vi "未命名 3.vi"() -> ()   [LabVIEW 2015]
uses:
  <vilib>/Utility/config.llb/Write Key (String).vi
  <vilib>/Utility/config.llb/Read Key (String).vi
  <vilib>/Utility/config.llb/NI_LVConfig.lvlib
panel:
  out "value":string caption="值"
  in  "停止":bool
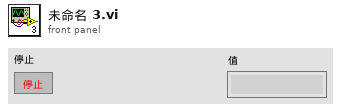
[diagram p1: front panel]
types:
  T1 = typedef "NI_LVConfig.lvlib/Config Data RefNum.ctl" = refnum<k1>
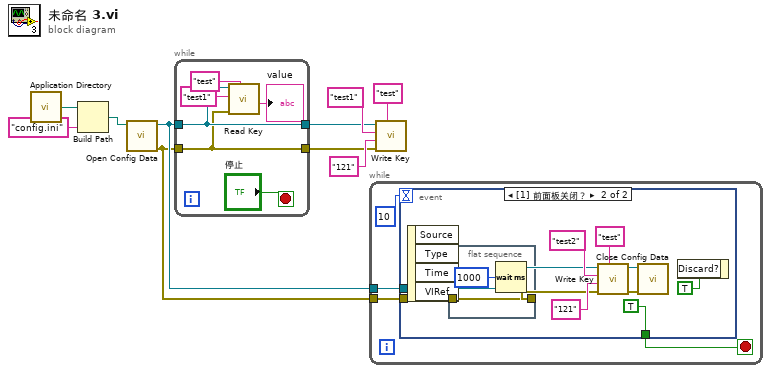
[diagram p0: block diagram]
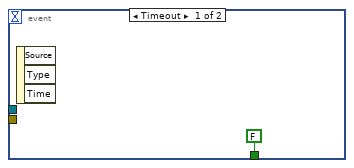
[diagram p2: hidden frame]
diagram:
  n1 = call <vilib>:"Application Directory.vi"() -> ("Application Directory"=w6:path)
  n2 = Build Path(base path=w6, name or relative path="config.ini" ("名称或相对路径")) -> (appended path=w5:path)
  n3 = call <vilib>:"Open Config Data.vi"("configuration file path"=w5) -> ("error out"=w1:errorcluster, "refnum"=w2:T1)  [unwired: 8 in, 1 out]
  n4 = while {
    tunnel: w2 -> [w15]
    tunnel: [w15] -> w4
    tunnel: w1 -> [w14]
    tunnel: [w14] -> w3
    stop <- "停止" stop-if-true
    n5 = call-poly <vilib>:"Read Key.vi"("section"="test", "error in (no error)"=w14, "key"="test1", "refnum"=w15) -> ("value"=→"value":string)  [unwired: 4 in, 3 out]
  }
  n6 = while {
    tunnel: w2 -> [w20]
    tunnel: w1 -> [w19]
    stop <- w18 stop-if-true
    n7 = event "事件结构" shown="[1] 前面板关闭？" {
      selector: _ -> [_ _]
      dyn-events: _ -> [_ _]
      timeout: 10 -> [_ _]
      tunnel: w20 -> [_ w28]
      tunnel: w19 -> [_ w24]
      tunnel: [FALSE TRUE] -> w18
      event Timeout {
        n8 = event-data() -> ()  [unwired: 1 in, 3 out]
      }
      event Panel Close? {
        n9 = event-data() -> ()  [unwired: 1 in, 4 out]
        n10 = flat-sequence {
          tunnel: w24 -> [w33]
          tunnel: [w33] -> w23
          frame #0 {
            n11 = Wait (ms)(milliseconds to wait=u32 1000 ("等待时间（毫秒）")) -> ()  [unwired: 1 out]
          }
        }
        n12 = call-poly <vilib>:"Write Key.vi"("section"="test", "error in (no error)"=w23, "value"="121" ("section"), "key"="test2", "refnum"=w28) -> ("error out"=w25:errorcluster, "refnum out"=w26:T1)  [unwired: 4 in, 1 out]
        n13 = call <vilib>:"Close Config Data.vi"("error in (no error)"=w25, "refnum"=w26) -> ()  [unwired: 8 in, 2 out]
        n14 = event-data("Discard?"=TRUE ("放弃？")) -> ()  [unwired: 1 in, 1 out]
      }
    }
  }
  n15 = call-poly <vilib>:"Write Key.vi"("section"="test", "error in (no error)"=w3, "value"="121" ("section"), "key"="test1", "refnum"=w4) -> ()  [unwired: 4 in, 3 out]
